vi "SCLN_GetMessageFromClient.vi"(0 "Server Name":string, 1 "error in (no error)":errorcluster) -> (2 "Index for Response":i32, 3 "Message":string, 4 "error out":errorcluster)   [LabVIEW 2015]
uses:
  SCLN_INT32_Select.ctl
  SCLN_RW_Select.ctl
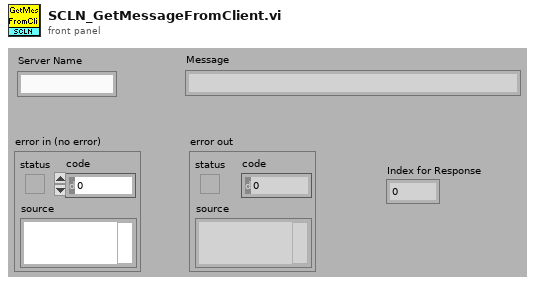
[diagram p1: front panel]
types:
  T1 = typedef "SCLN_RW_Select.ctl" = enum16{"Read", "Write"}
  T2 = typedef "SCLN_INT32_Select.ctl" = enum16{"Max_Servers", "Max_Clients", "Total_Servers", "Total_Clients"}
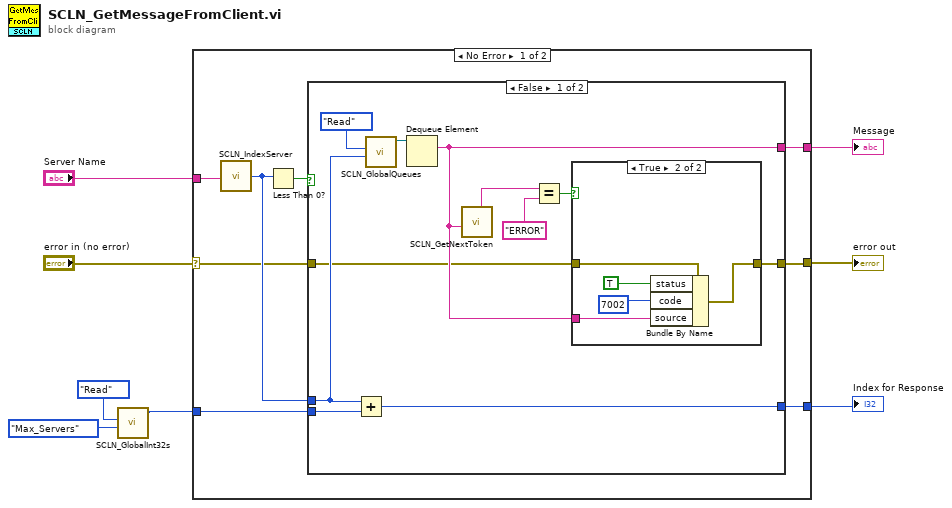
[diagram p0: block diagram]
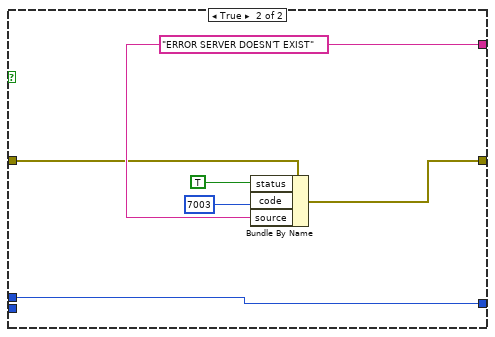
[diagram p3: hidden frame]
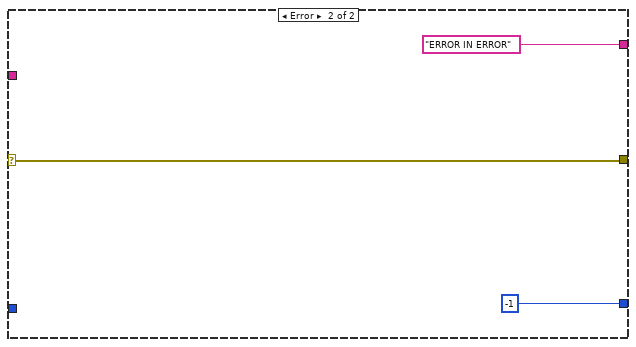
[diagram p4: hidden frame]
diagram:
  n1 = call "SCLN_GlobalInt32s.vi"("Element"=SCLN_INT32_Select."Max_Servers" ("GBL_INT32"), "Operation"=SCLN_RW_Select."Read" ("GBL_RW")) -> ("Read Value"=w1:i32)  [unwired: 2 in, 1 out]
  n2 = case shown="No Error" "error in (no error)" {
    selector: "error in (no error)" -> [w9 w40]
    tunnel: [w12 -1] -> w8
    tunnel: [w14 "ERROR IN ERROR"] -> w7
    tunnel: "Server Name" -> [w16 _]
    tunnel: [w11 w40] -> w4
    tunnel: w1 -> [w10 _]
    frame No Error {
      n3 = call "SCLN_IndexServer.vi"("Server Name"=w16) -> ("Index"=w13:i32)
      n4 = Less Than 0?(x=w13) -> (x < 0?=w15:bool)
      n5 = case shown="False" w15 {
        tunnel: [w18 w36] -> w14
        tunnel: w13 -> [w26 w39]
        tunnel: [w25 w39] -> w12
        tunnel: [w21 w35] -> w11
        tunnel: w10 -> [w20 _]
        tunnel: w9 -> [w17 w34]
        frame False {
          n6 = Add(x=w26, y=w20) -> (x+y=w25:i32)
          n7 = call "SCLN_GlobalQueues.vi"("Element"=w26, "Operation"=SCLN_RW_Select."Read" ("GBL_RW")) -> ("Read QueueID"=w19:refnum<queue>)  [unwired: 6 in, 1 out]
          n8 = Dequeue Element(queue=w19) -> (element=w18:string)  [unwired: 2 in, 3 out]
          n9 = call "SCLN_GetNextToken.vi"("Input string"=w18) -> ("Token"=w23:string)  [unwired: 4 in, 1 out]
          n10 = Equal?(x=w23, y="ERROR") -> (x = y?=w22:bool)
          n11 = case shown="True" w22 {
            tunnel: w17 -> [w28 w33]
            tunnel: [w28 w30] -> w21
            tunnel: w18 -> [_ w29]
            frame False {
            }
            frame True {
              n12 = Bundle By Name(cluster=w33, "status"=TRUE, "code"=7002, "source"=w29) -> (w30:errorcluster)
            }
          }
        }
        frame True {
          w36 = "ERROR SERVER DOESN'T EXIST"
          n13 = Bundle By Name(cluster=w34, "status"=TRUE, "code"=7003, "source"=w36) -> (w35:errorcluster)
        }
      }
    }
    frame Error {
    }
  }
  "Message" <- w7
  "error out" <- w4
  "Index for Response" <- w8
